vi "Action - TDMS Writer.vi"(8 "error in":errorcluster, 11 "tdms file ref":refnum<k34>) -> (0 "error out":errorcluster)   [LabVIEW 2021, in "XNET-CAN-Signal-Logger.lvlib"]
uses:
  XNET-CAN-Signal-Logger.lvlib
  Typedef/Def-Data Queue Type.ctl
  Typedef/Def-GSTOP.ctl
  Global Variables.vi
  <userlib>/_NEVSTOP/GlobalStop/_gStop.vi
  <userlib>/_NEVSTOP/GlobalStop/GSTOP.lvlib
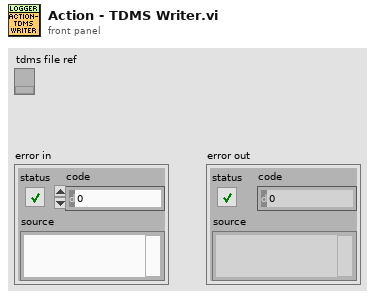
[diagram p1: front panel]
types:
  T1 = typedef "XNET-CAN-Signal-Logger.lvlib/Def-GSTOP.ctl" = enum16{"Writer", "Readers"}
  T2 = typedef "XNET-CAN-Signal-Logger.lvlib/Def-Data Queue Type.ctl" = cluster{"PackageID":i32, "Data":waveform(dbl)[]}
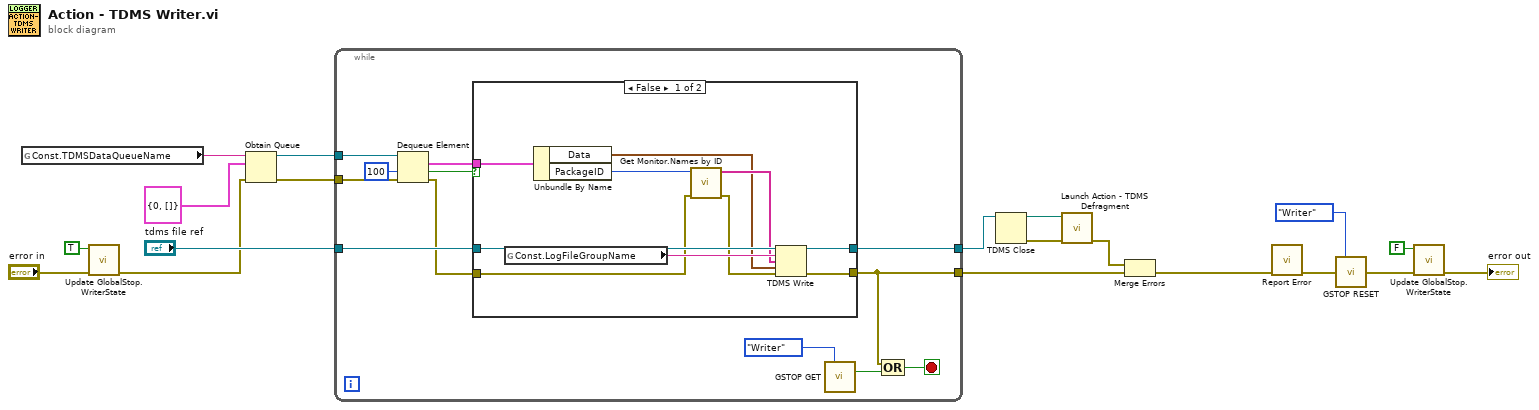
[diagram p0: block diagram]
diagram:
  n1 = global read "Global Variables.vi" "Const.TDMSDataQueueName"() -> (w19:string)
  n2 = call "Update GlobalStop.WriterState.vi"("error in"="error in", "RunState"=TRUE) -> ("error out"=w3:errorcluster)  [unwired: 9 in]
  n3 = Obtain Queue(name (unnamed)=w19, element data type=T2 {"PackageID"=0, "Data"=[]} ("Data Queue Type"), error in (no error)=w3) -> (queue out=w17:refnum<queue>, error out=w16:errorcluster)  [unwired: 2 in, 1 out]
  n4 = while {
    tunnel: [w31] -> w11
    tunnel: "tdms file ref" -> [w30]
    tunnel: [w22] -> w12
    tunnel: w17 -> [w29]
    tunnel: w16 -> [w24]
    stop <- w23 stop-if-true
    n5 = Dequeue Element(queue=w29, timeout in ms (-1)=100, error in (no error)=w24) -> (element=w28:T2, timed out?=w25:bool, error out=w27:errorcluster)  [unwired: 1 out]
    n6 = case shown="False" w25 {
      tunnel: [w41 w43] -> w31
      tunnel: w30 -> [w40 w43]
      tunnel: [w39 w42] -> w22
      tunnel: w28 -> [w37 _]
      tunnel: w27 -> [w35 w42]
      frame False {
        n7 = global read "Global Variables.vi" "Const.LogFileGroupName"() -> (w38:string)
        n8 = Unbundle By Name(w37) -> ("Data"=w32:waveform(dbl)[], "PackageID"=w36:i32)
        n9 = call "Get Monitor.Names by ID.vi"("error in"=w35, "PackageID"=w36) -> ("error out"=w34:errorcluster, "Signal Names"=w33:string[])  [unwired: 8 in]
        n10 = TDMS Write(0:w40, 5:w38, 7:w33, 9:w32, 11:w34) -> (4:w41:refnum<k34>, 15:w39:errorcluster)  [unwired: 1 in, 2 out]
      }
      frame True {
      }
    }
    n11 = call <userlib>:"GSTOP GET.vi"("index(-1 for All)"=Def-GSTOP."Writer" ("GSTOP")) -> ("stop"=w21:bool)  [unwired: 13 in, 1 out]
    n12 = Compound Arithmetic op=OR(w22, w21) -> (w23:bool)
  }
  n13 = TDMS Close(11:w11) -> (0:w14:errorcluster, 3:w7:path)  [unwired: 1 in]
  n14 = call "Launch Action - TDMS Defragment.vi"("error in (no error)"=w14, "file path"=w7) -> ("error out"=w8:errorcluster)  [unwired: 9 in]
  n15 = Merge Errors(w8, w12) -> (w13:errorcluster)
  n16 = call "Report Error.vi"("error in (no error)"=w13) -> ("error out"=w15:errorcluster)  [unwired: 10 in]
  n17 = call <userlib>:"GSTOP RESET.vi"("index(-1 for All)"=Def-GSTOP."Writer" ("GSTOP"), "error in (no error)"=w15) -> ("error out"=w2:errorcluster)  [unwired: 13 in]
  n18 = call "Update GlobalStop.WriterState.vi"("error in"=w2, "RunState"=FALSE) -> ("error out"=→"error out":errorcluster)  [unwired: 9 in]
